vi "Is Overhaul.vi"(8 "overhaul in":bool, 9 "goal node in":refnum<data-value>, 10 "current node in":refnum<data-value>, 11 "AD* in":refnum<class "NI_Robotics_AnytimeDStar.lvclass">) -> (0 "overhaul out":bool, 1 "goal node out":refnum<data-value>, 2 "current node out":refnum<data-value>, 3 "AD* out":refnum<class "NI_Robotics_AnytimeDStar.lvclass">)   [LabVIEW 2017, in "NI_Robotics_AnytimeDStar.lvclass"]
uses:
  <vilib>/robotics/Navigation/Anytime D Star/NI_Robotics_AnytimeDStar.lvclass
  <vilib>/robotics/Navigation/shared/MapNode/AbstractDstarNode/NI_Robotics_AbstractDstarNode.lvclass
  <vilib>/robotics/Navigation/Anytime D Star/NI_Robotics_AnytimeDStar.lvclass/NI_Robotics_AnytimeDStar.ctl
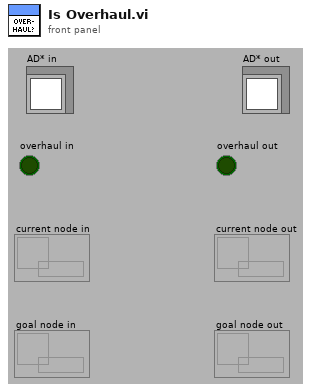
[diagram p1: front panel]
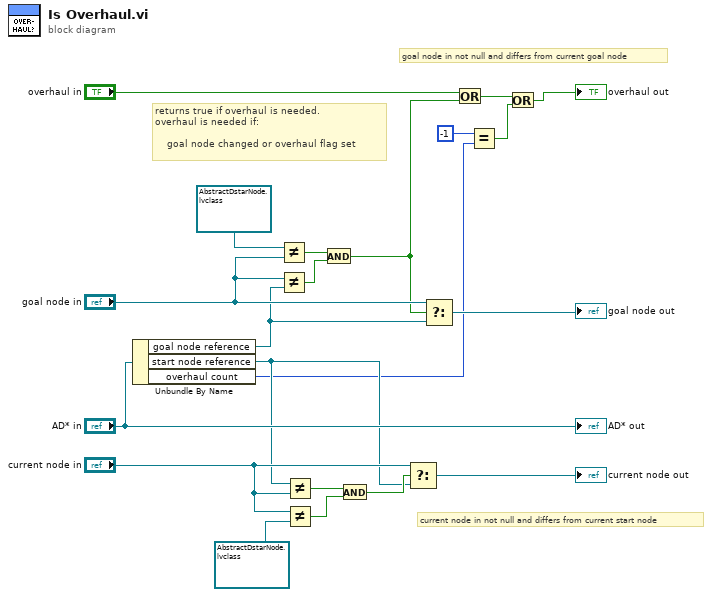
[diagram p0: block diagram]
diagram:
  # "returns true if overhaul is needed.\noverhaul is needed if:\n\n    goal node changed or overhaul flag set"
  # "current node in not null and differs from current start node"
  # "goal node in not null and differs from current goal node"
  n1 = Unbundle By Name("AD* in") -> ("goal node reference"=w7:refnum<data-value>, "start node reference"=w14:refnum<data-value>, "overhaul count"=w5:i32)
  n2 = Not Equal?(x=refnum<data-value> refnum ("node in"), y="goal node in") -> (x != y?=w11:bool)
  n3 = Not Equal?(x="goal node in", y=w7) -> (x != y?=w10:bool)
  n4 = Not Equal?(x=w14, y="current node in") -> (x != y?=w17:bool)
  n5 = Not Equal?(x="current node in", y=refnum<data-value> refnum ("node in")) -> (x != y?=w18:bool)
  n6 = And(x=w11, y=w10) -> (x .and. y?=w6:bool)
  n7 = And(x=w17, y=w18) -> (x .and. y?=w16:bool)
  n8 = Select(t="current node in", s=w16, f=w14) -> (s? t:f=→"current node out":refnum<data-value>)
  n9 = Select(t="goal node in", s=w6, f=w7) -> (s? t:f=→"goal node out":refnum<data-value>)
  n10 = Or(x="overhaul in", y=w6) -> (x .or. y?=w3:bool)
  n11 = Equal?(x=-1, y=w5) -> (x = y?=w2:bool)
  n12 = Or(x=w3, y=w2) -> (x .or. y?=→"overhaul out":bool)
  "AD* out" <- "AD* in"
